vi "OverlayLandmark.vi"(8 "error in (no error)":errorcluster, 10 ".NET Refnum in":refnum<k24>, 11 "New Image":T1) -> (0 "error out":errorcluster, 3 "Image Out":T1)   [LabVIEW 2017]
uses:
  <vilib>/vision/Image Controls.llb/IMAQ Image.ctl
  ctl/Point.ctl
  FaceRecognition.lvclass
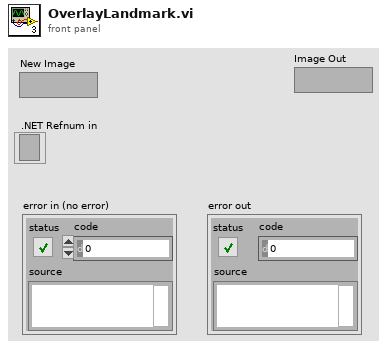
[diagram p1: front panel]
types:
  T1 = typedef "IMAQ Image.ctl" = refnum<image>
  T2 = typedef "FaceRecognitionDotNet.lvlib/FaceRecognition.lvclass/FacePart.ctl" = i32
  T3 = typedef "FaceRecognitionDotNet.lvlib/FaceRecognition.lvclass/Point.ctl" = cluster{"X":sgl, "Y":sgl}
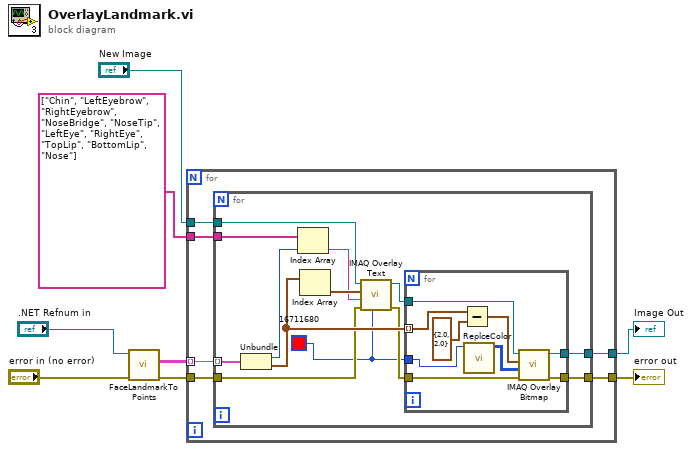
[diagram p0: block diagram]
diagram:
  n1 = call "FaceLandmarkToPoints.vi"("error in (no error)"="error in (no error)", "FaceLandmark"=".NET Refnum in") -> ("error out"=w7:errorcluster, "FaceLandmarkArray"=w5:cluster{"item":T2, T3[]}[][])  [unwired: 8 in]
  n2 = for {
    tunnel: w5 -> [w14] mode=indexing
    tunnel: "New Image" -> [w13]
    tunnel: w7 -> [w12]
    tunnel: [w11] -> w3
    tunnel: [w10] -> w2
    tunnel: string[] ["Chin", "LeftEyebrow", "RightEyebrow", "NoseBridge", "NoseTip", "LeftEye", "RightEye", "TopLip", "BottomLip", "Nose"] -> [w9]
    n3 = for {
      tunnel: w14 -> [w27] mode=indexing
      tunnel: w13 -> [w24]
      tunnel: w12 -> [w17]
      tunnel: [w25] -> w11
      tunnel: [w26] -> w10
      tunnel: w9 -> [w19]
      w15 = u32 16711680
      n4 = Unbundle(w27) -> ("item"=w20:T2, w22:T3[])
      n5 = Index Array(array=w19, index=w20) -> (element=w18:string)
      n6 = Index Array(array=w22) -> (element=w21:T3)  [unwired: 1 in]
      n7 = call "IMAQ Overlay Text"("Text Color (black)"=w15, "error in (no error)"=w17, "String"=w18, "Origin"=w21, "Image"=w24) -> ("error out"=w16:errorcluster, "Image Out"=w23:T1)  [unwired: 5 in]
      n8 = for {
        tunnel: w22 -> [w35] mode=indexing
        tunnel: w15 -> [w28]
        tunnel: w23 -> [w32]
        tunnel: [w31] -> w26
        tunnel: w16 -> [w30]
        tunnel: [w29] -> w25
        n9 = Subtract(x=w35, y=T3 {"X"=2.0, "Y"=2.0}) -> (x-y=w33:T3)
        n10 = call "ReplceColor.vi"("Color Box"=w28) -> ("Array"=w36:u32[][])  [unwired: 10 in]
        n11 = call "IMAQ Overlay Bitmap"("error in (no error)"=w30, "Bitmap"=w36, "Top Left Point"=w33, "Image"=w32) -> ("error out"=w29:errorcluster, "Image Out"=w31:T1)  [unwired: 6 in]
      }
    }
  }
  "error out" <- w3
  "Image Out" <- w2
